vi "Flow_Selection_2.vi"(9 "Linearized Temperature":sgl, 10 "Flow":dbl, 11 "Pressure Transducer 2":enum32{"Druck ", "FUJI ", "Impress"}(ring)) -> (1 "Flow rate g/s":dbl, 2 "Flow rate l/min":dbl)   [LabVIEW 2014]
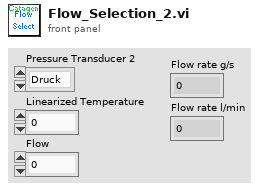
[diagram p1: front panel]
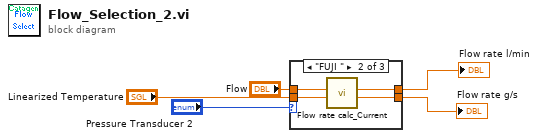
[diagram p0: block diagram]
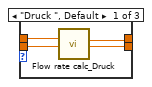
[diagram p2: hidden frame]
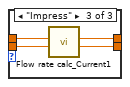
[diagram p3: hidden frame]
diagram:
  n1 = case shown="\"FUJI \"" "Pressure Transducer 2" {
    tunnel: "Flow" -> [w9 w13 w17]
    tunnel: [w7 w11 w16] -> w2
    tunnel: "Linearized Temperature" -> [w8 w12 w15]
    tunnel: [w6 w10 w14] -> w1
    frame "Druck ", Default {
      n2 = call "Flow rate calc_Druck.vi"("T venturi"=w8, "P venturi"=w9) -> ("Flow rate g/s"=w7:dbl, "Flow rate l/min"=w6:dbl)  [unwired: 8 in]
    }
    frame "FUJI " {
      n3 = call "Flow rate calc_Current.vi"("T venturi"=w12, "P venturi"=w13) -> ("Flow rate g/s"=w11:dbl, "Flow rate l/min"=w10:dbl)  [unwired: 8 in]
    }
    frame "Impress" {
      n4 = call "Flow rate calc_Current1.vi"("T venturi"=w15, "P venturi"=w17) -> ("Flow rate g/s"=w16:dbl, "Flow rate l/min"=w14:dbl)  [unwired: 8 in]
    }
  }
  "Flow rate g/s" <- w2
  "Flow rate l/min" <- w1
